vi "CircularBuffer.TestLauncher.vi"() -> ()   [LabVIEW 2016, in "CircularBuffer.lvclass"]
doc: "JKI State Machine Objects (SMO) 1.0.0.5\nJKI - JKI\nCopyright (c) 2016, JKI"
uses:
  CircularBuffer.lvclass
  <vilib>/JKI/JKI SMO/SMO/SMO.lvclass
  <vilib>/JKI/JKI SMO/SMO/Typedefs/SMOState --Enum.ctl
  C:/Program Files (x86)/National Instruments/LabVIEW 2016/vi.lib/JKI/JKI SMO/SMO/SMO.lvclass
panel:
  out "newestElementIndex":i32
  in  "Offset":u8=50
  in  "Generate":bool
  out "index":i32
  out "data":u8
  out "BufferSize":i32
  out "State":T1
  out "error out":errorcluster
  in  "Stop":bool
  # "Circular Buffer Test Launcher"
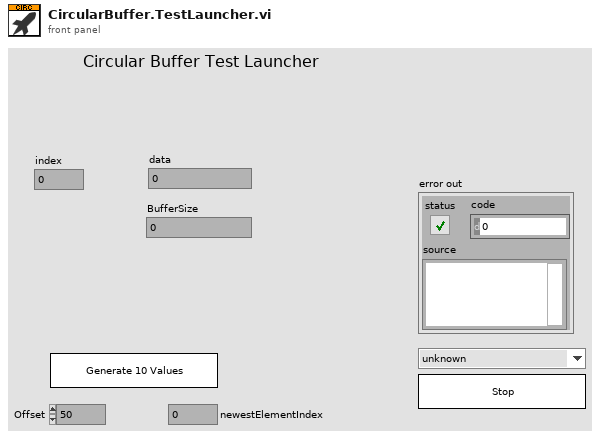
[diagram p1: front panel]
types:
  T1 = typedef "SMO.lvclass/SMOState --Enum.ctl" = enum16{"unknown", "Created", "Started", "Stopped"}
  T2 = typedef "CircularBuffer.lvclass/PublicEvents--Cluster.ctl" = cluster{"Buffer Resize Event":refnum<user-event>}
  T3 = typedef "SMO.lvclass/Public Events.ctl" = cluster{"Error":refnum<user-event>, "State":refnum<user-event>}
  T4 = cluster{"Event Registration Refnum":refnum<event-registration>}
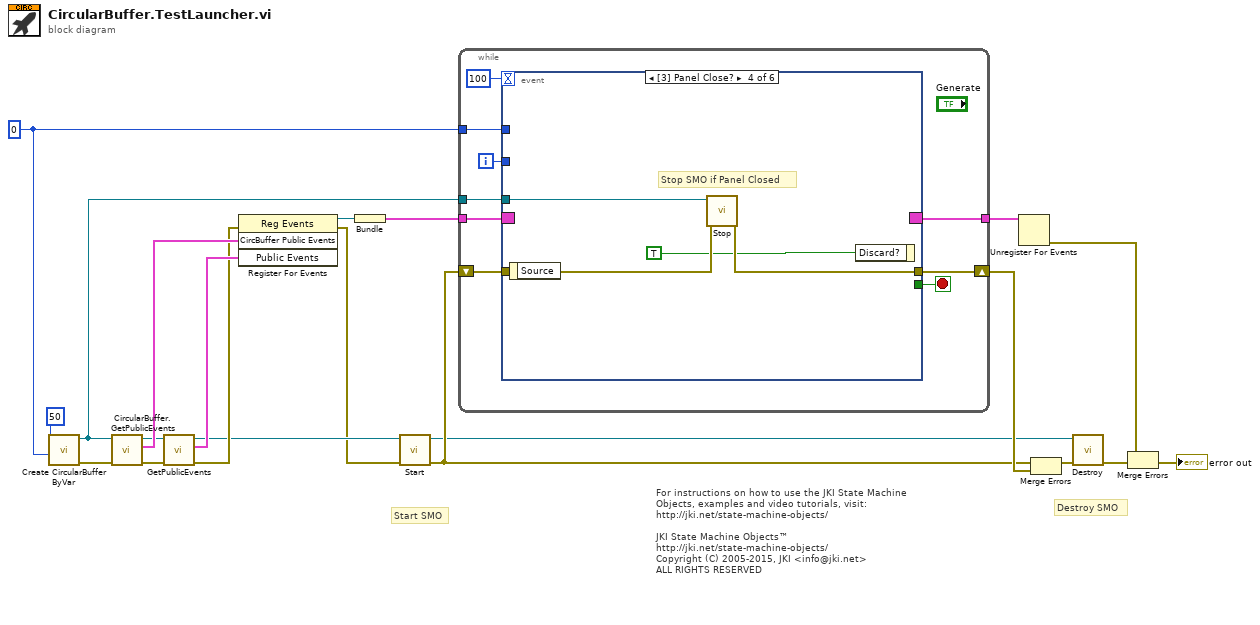
[diagram p0: block diagram]
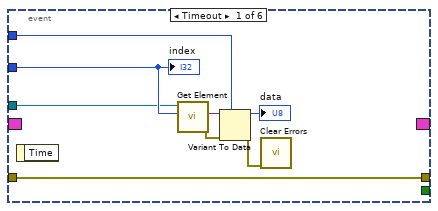
[diagram p2: hidden frame]
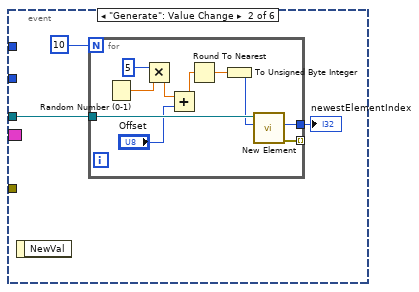
[diagram p3: hidden frame]
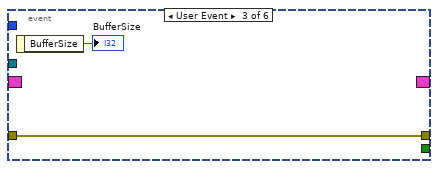
[diagram p4: hidden frame]
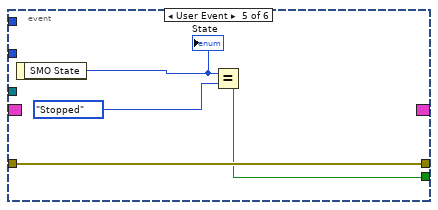
[diagram p5: hidden frame]
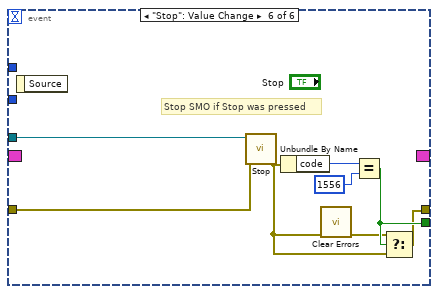
[diagram p6: hidden frame]
diagram:
  w1 = u8 0 ("value")
  # "For instructions on how to use the JKI State Machine Objects, examples and video tutorials, visit:\nhttp://jki.net/state-machine-objects/\n\nJKI State Machine Objects™\nhttp://jki.net/state-machine-objects/\nCopyright (C) 2005-2015, JKI <info@jki.net>\nALL RIGHTS RESERVED"
  # "Start SMO"
  # "Destroy SMO"
  n1 = call "Create CircularBuffer ByVar.vi"("Type"=w1, "BufferSize"=u32 50) -> ("error out"=w2:errorcluster, "CircularBuffer out"=w3:refnum<class "CircularBuffer.lvclass">)  [unwired: 7 in, 1 out]
  n2 = call "CircularBuffer.GetPublicEvents.vi"("error in (no error)"=w2, "CircularBuffer"=w3) -> ("error out"=w11:errorcluster, "CircBuffer Public Events"=w14:T2, "CircularBuffer out"=w12:refnum<class "CircularBuffer.lvclass">)  [unwired: 7 in]
  n3 = call <vilib>:"GetPublicEvents.vi"("error in (no error)"=w11, "SMO"=w12) -> ("error out"=w9:errorcluster, "Public Events"=w10:T3, "SMO out"=w6:refnum<class "CircularBuffer.lvclass">)  [unwired: 7 in]
  n4 = register-events(error in=w9, w14, w10) -> (reference out=w13:refnum<event-registration>, error out=w5:errorcluster)  [unwired: 1 in]
  n5 = Bundle("Event Registration Refnum"=w13) -> (w20:T4)  [unwired: 1 in]
  n6 = call <vilib>:"Start.vi"("error in (no error)"=w5, "SMO"=w6) -> ("error out"=w15:errorcluster, "SMO out"=w7:refnum<class "CircularBuffer.lvclass">)  [unwired: 8 in]
  n7 = while {
    shift-right: [w29] -> w19
    shift-left: w15 -> [w28]
    tunnel: w20 -> [w27]
    tunnel: [w26] -> w21
    tunnel: w3 -> [w25]
    tunnel: w1 -> [w23]
    i -> [w22]
    stop <- w30 stop-if-true
    n8 = event shown="[3] Panel Close?" {
      selector: w27 -> [_ _ _ _ _ _]
      dyn-events: [_ _ _ _ _ _] -> w26
      timeout: 100 -> [_ _ _ _ _ _]
      tunnel: [_ _ _ _ w58 w65] -> w30
      tunnel: w25 -> [w32 w40 _ w57 _ w69]
      tunnel: [w38 _ w53 w56 w61 w64] -> w29
      tunnel: w28 -> [w38 _ w53 w55 w61 w68]
      tunnel: w23 -> [w31 _ _ _ _ _]
      tunnel: w22 -> [w33 _ _ _ _ _]
      event Timeout {
        n9 = event-data() -> ()  [unwired: 1 in, 1 out]
        n10 = call "Get Element.vi"("GetElement (-1: Current)"=w33, "CircularBuffer"=w32) -> ("error out"=w36:errorcluster, "Element"=w37:variant)  [unwired: 7 in, 1 out]
        n11 = Variant To Data(error in=w36, type=w31, Variant=w37) -> (data=→"data":u8, error out=w35:errorcluster)
        n12 = call <vilib>:"Clear Errors.vi"("error in (no error)"=w35) -> ()  [unwired: 5 in, 2 out]
        "index" <- w33
      }
      event "Generate": Value Change {
        n13 = event-data() -> ()  [unwired: 1 in, 1 out]
        n14 = for {
          N: u32 10 ("# Data to generate") -> [_]
          tunnel: w40 -> [w48]
          tunnel: [w46] -> _ mode=indexing
          tunnel: [w42] -> w39
          n15 = Random Number (0-1)() -> (number: 0 to 1=w50:dbl)
          n16 = Multiply(x=u8 5 ("Amplitude"), y=w50) -> (x*y=w44:dbl)
          n17 = Add(x=w44, y="Offset") -> (x+y=w43:dbl)
          n18 = Round To Nearest(number=w43) -> (nearest integer value=w49:dbl)
          n19 = To Unsigned Byte Integer(number=w49) -> (unsigned 8bit integer=w47:u8)
          n20 = call "New Element.vi"("Element"=w47, "CircularBuffer"=w48) -> ("error out"=w46:errorcluster, "newElementIndex"=w42:i32)  [unwired: 7 in, 1 out]
        }
        "newestElementIndex" <- w39
      }
      event User Event {
        n21 = event-data() -> ("BufferSize"=→"BufferSize":i32)  [unwired: 1 in]
      }
      event Panel Close? {
        # "Stop SMO if Panel Closed"
        n22 = event-data() -> ()  [unwired: 1 in, 1 out]
        n23 = call <vilib>:"Stop.vi"("error in (no error)"=w55, "SMO"=w57) -> ("error out"=w56:errorcluster)  [unwired: 8 in, 1 out]
        n24 = event-data("Discard?"=TRUE ("OK")) -> ()  [unwired: 1 in, 1 out]
      }
      event User Event {
        n25 = event-data() -> ("SMO State"=w60:T1)  [unwired: 1 in]
        "State" <- w60
        n26 = Equal?(x=w60, y=SMOState_--Enum."Stopped") -> (x = y?=w58:bool)
      }
      event "Stop": Value Change {
        # "Stop SMO if Stop was pressed"
        n27 = event-data() -> ()  [unwired: 1 in, 1 out]
        n28 = call <vilib>:"Stop.vi"("error in (no error)"=w68, "SMO"=w69) -> ("error out"=w63:errorcluster)  [unwired: 8 in, 1 out]
        n29 = Unbundle By Name(w63) -> ("code"=w67:i32)
        n30 = call <vilib>:"Clear Errors.vi"("error in (no error)"=w63) -> ("error out"=w62:errorcluster)  [unwired: 5 in, 1 out]
        n31 = Equal?(x=w67, y=1556 ("specific error code to clear (0: all)")) -> (x = y?=w65:bool)
        n32 = Select(t=w62, s=w65, f=w63) -> (s? t:f=w64:errorcluster)
      }
    }
  }
  n33 = Unregister For Events(event registration refnum=w21) -> (error out=w18:errorcluster)  [unwired: 1 in]
  n34 = Merge Errors(w15, w19) -> (w8:errorcluster)
  n35 = call <vilib>:"Destroy.vi"("error in (no error)"=w8, "SMO"=w7) -> ("error out"=w16:errorcluster)  [unwired: 9 in]
  n36 = Merge Errors(w18, w16) -> (→"error out":errorcluster)
